vi "Get Array Value at Index - Null.vi"(8 "error in (no error)":errorcluster, 10 "Index":i32, 11 "JSON Tree In (JSON Array)":variant) -> (0 "error out":errorcluster, 1 "is JSON Null?":bool, 2 "JSON Null Value":variant, 3 "JSON Tree Out Passthrough":variant)   [LabVIEW 2011, in "i3-json.lvlib"]
doc: "Use this template to build a VI to use as a subVI."
uses:
  i3-json.lvlib
  JSON Types/JSON Type.ctl
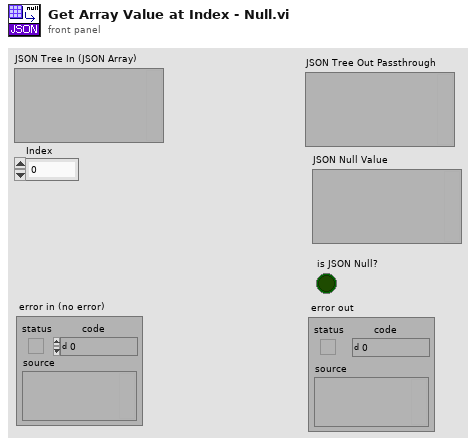
[diagram p1: front panel]
types:
  T1 = typedef "i3-json.lvlib/JSON Type.ctl" = enum8{"JSON Compatible", "JSON Array", "JSON Object", "JSON Null", "Double", "String", "Boolean", "Unknown"}
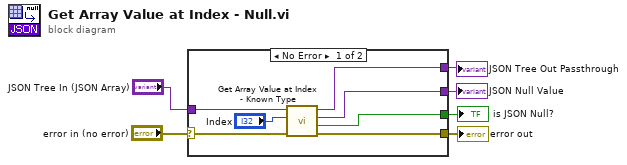
[diagram p0: block diagram]
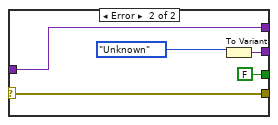
[diagram p2: hidden frame]
diagram:
  n1 = case shown="No Error" "error in (no error)" {
    selector: "error in (no error)" -> [w10 w18]
    tunnel: [w9 w18] -> w5
    tunnel: "JSON Tree In (JSON Array)" -> [w13 w17]
    tunnel: [w11 w17] -> w3
    tunnel: [w8 FALSE ("is JSON Null?")] -> w2
    tunnel: [w7 w16] -> w1
    frame No Error {
      n2 = call "Get Array Value at Index - Known Type.vi"("error in (no error)"=w10, "Index"="Index", "JSON Tree In (JSON Array)"=w13) -> ("error out"=w9:errorcluster, "is JSON Null?"=w8:bool, "Value"=w7:variant, "JSON Tree Out Passthrough"=w11:variant)  [unwired: 3 in, 2 out]
    }
    frame Error {
      n3 = To Variant(anything=JSON_Type."Unknown" ("JSON Type")) -> (Variant=w16:variant)
    }
  }
  "error out" <- w5
  "JSON Tree Out Passthrough" <- w3
  "is JSON Null?" <- w2
  "JSON Null Value" <- w1
